vi "sio iqueue.vi"(11 "port":i32) -> (1 "len":i32, 2 "not empty":bool, 3 "port":i32)   [LabVIEW 2015, in "PCOMM.lvlib"]
doc: "long WINAPI sio_iqueue(int port);\n接收到的数据量不为0，bool 类型 返回true"
uses:
  PCOMM.lvlib
  PCOMM.DLL
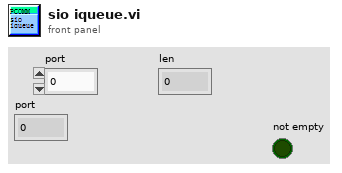
[diagram p1: front panel]
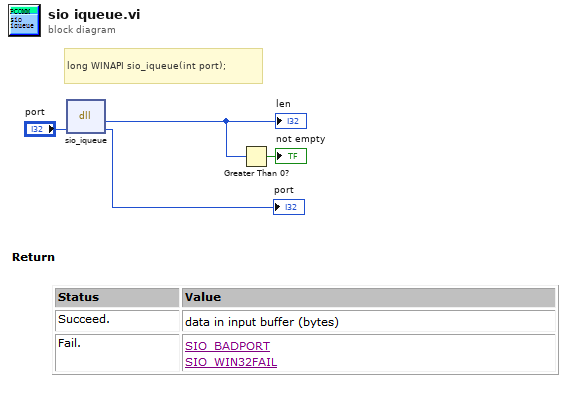
[diagram p0: block diagram]
diagram:
  # "long WINAPI sio_iqueue(int port);"
  n1 = dll-call lib="PTH2Yabs EDesktopLabview串口助手串口助手2.0Ing10_v3.2.0libpcommPCOMM.*" fn="sio_iqueue"("port"="port") -> (w3:i32, "port"=→"port":i32)  [unwired: 3 in, 2 out]
  "len" <- w3
  n2 = Greater Than 0?(x=w3) -> (x > 0?=→"not empty":bool)
